vi "Group Services.vi"(8 "error in":errorcluster, 11 "gRPC Method Parameters":T1[](array[typedef])) -> (0 "error out":errorcluster, 3 "Service Methods":cluster{"gRPC Method Parameters":T1[]}[](array[cluster]))   [LabVIEW 2019, in "gRPC Template Creation Utility.lvlib"]
uses:
  gRPC Template Creation Utility.lvlib
  TypeDefs/RPC Method Parameters.ctl
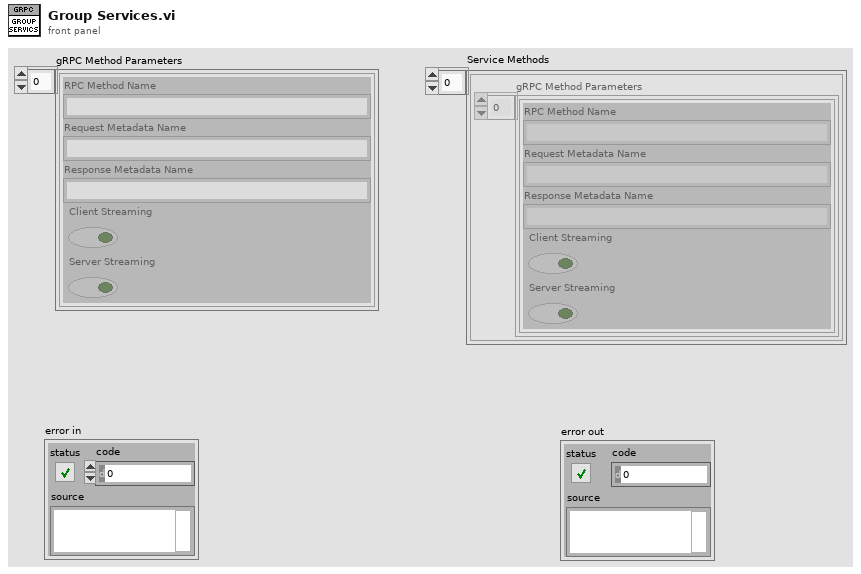
[diagram p1: front panel]
types:
  T1 = typedef "gRPC Template Creation Utility.lvlib/RPC Method Parameters.ctl" = cluster{"RPC Method Name":string, "Request Metadata Name":string, "Response Metadata Name":string, "Client Streaming":bool, "Server Streaming":bool}
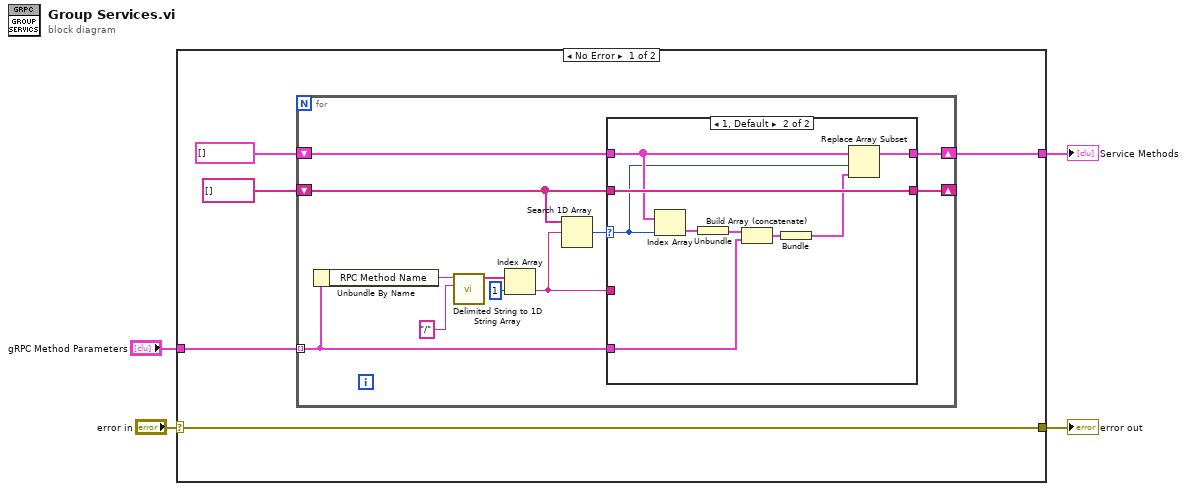
[diagram p0: block diagram]
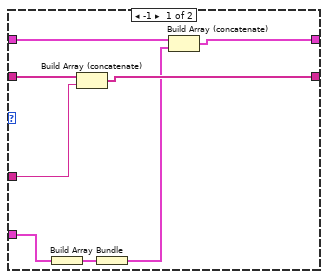
[diagram p2: hidden frame]
diagram:
  n1 = case shown="No Error" "error in" {
    selector: "error in" -> [w5 w38]
    tunnel: [w5 w38] -> w4
    tunnel: "gRPC Method Parameters" -> [w9 _]
    tunnel: [w7 _] -> w1
    frame No Error {
      n2 = for {
        tunnel: w9 -> [w11] mode=indexing
        shift-right: [w13] -> w7
        shift-left: cluster{"gRPC Method Parameters":T1[]}[] [] ("Service Methods") -> [w14]
        shift-right: [w15] -> _
        shift-left: string[] [] -> [w16]
        n3 = Unbundle By Name(w11) -> ("RPC Method Name"=w20:string)
        n4 = call <vilib>:"Delimited String to 1D String Array.vi"("delimiter"="/", "delimited string"=w20) -> ("string array"=w18:string[])  [unwired: 9 in]
        n5 = Index Array(array=w18, index=1) -> (element=w12:string)
        n6 = Search 1D Array(1D array=w16, element=w12) -> (index of element=w17:i32)  [unwired: 1 in]
        n7 = case shown="1, Default" w17 {
          selector: w17 -> [_ w29]
          tunnel: w16 -> [w28 w37]
          tunnel: [w27 w37] -> w15
          tunnel: w14 -> [w25 w36]
          tunnel: [w21 w31] -> w13
          tunnel: w12 -> [w26 _]
          tunnel: w11 -> [w24 w33]
          frame -1 {
            n8 = Build Array(w24) -> (w23:T1[])
            n9 = Build Array (concatenate)(w28, w26) -> (w27:string[])
            n10 = Bundle(w23) -> (w22:cluster{T1[]})  [unwired: 1 in]
            n11 = Build Array (concatenate)(w25, w22) -> (w21:cluster{"gRPC Method Parameters":T1[]}[])
          }
          frame 1, Default {
            n12 = Index Array(array=w36, index=w29) -> (element=w35:cluster{"gRPC Method Parameters":T1[]})
            n13 = Unbundle(w35) -> ("gRPC Method Parameters"=w34:T1[])
            n14 = Build Array (concatenate)(w34, w33) -> (w32:T1[])
            n15 = Bundle(w32) -> (w30:cluster{T1[]})  [unwired: 1 in]
            n16 = Replace Array Subset(array=w36, new element=w30, index=w29) -> (w31:cluster{"gRPC Method Parameters":T1[]}[])
          }
        }
      }
    }
    frame Error {
    }
  }
  "error out" <- w4
  "Service Methods" <- w1
